vi "PID Active_Buffer_Bool_VIG.vi"(7 "Operation":enum16{"get data", "set data", "initialize"}(ring)=enum."set data", 8 "error in":errorcluster, 11 "Boolean":bool) -> (0 "error out":errorcluster, 3 "Boolean 2":bool)   [LabVIEW 2018]
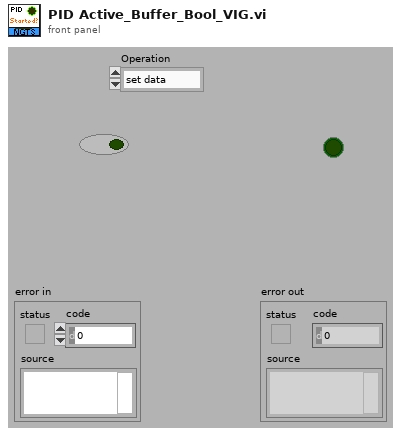
[diagram p1: front panel]
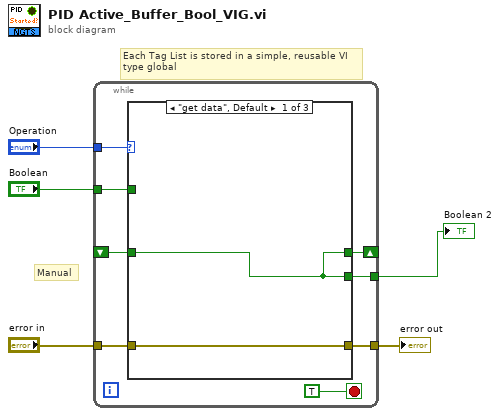
[diagram p0: block diagram]
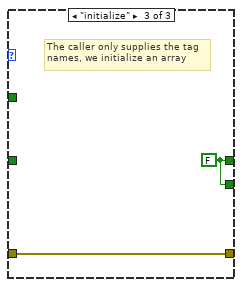
[diagram p3: hidden frame]
diagram:
  # "Manual"
  # "Each Tag List is stored in a simple, reusable VI\ntype global"
  n1 = while {
    tunnel: "Operation" -> [w13]
    tunnel: "Boolean" -> [w11]
    tunnel: "error in" -> [w10]
    tunnel: [w9] -> w2
    shift-right: [w8] -> _
    shift-left: _ -> [w7]
    tunnel: [w6] -> w1
    stop <- TRUE stop-if-true
    n2 = case shown="\"get data\", Default" w13 {
      tunnel: w11 -> [_ w16 _]
      tunnel: w10 -> [w15 w17 w19]
      tunnel: [w15 w17 w19] -> w9
      tunnel: [w14 w16 w18] -> w8
      tunnel: w7 -> [w14 _ _]
      tunnel: [w14 w16 w18] -> w6
      frame "get data", Default {
      }
      frame "set data" {
      }
      frame "initialize" {
        w18 = FALSE ("Boolean")
        # "The caller only supplies the tag\nnames, we initialize an array"
      }
    }
  }
  "error out" <- w2
  "Boolean 2" <- w1
